vi "Close TDMS File.vi"(8 "error in (no error)":errorcluster caption="错误输入（无错误）", 11 "Log File":refnum<k34> caption="记录文件") -> (0 "error out":errorcluster caption="错误输出", 3 "file path":path caption="记录文件路径")   [LabVIEW 2015]
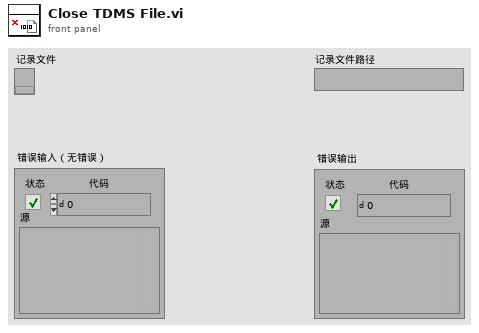
[diagram p1: front panel]
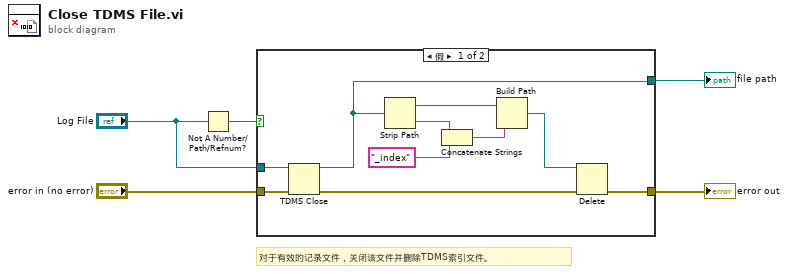
[diagram p0: block diagram]
diagram:
  # "对于有效的记录文件，关闭该文件并删除TDMS索引文件。"
  n1 = Not A Number/Path/Refnum?(number/path/refnum="Log File") -> (NaN/Path/Refnum?=w4:bool)
  n2 = case shown="假" w4 {
    tunnel: [w14 w16] -> w2
    tunnel: "error in (no error)" -> [w8 w16]
    tunnel: "Log File" -> [w7 _]
    tunnel: [w6 _] -> w1
    frame False {
      n3 = TDMS Close(8:w8, 11:w7) -> (0:w9:errorcluster, 3:w6:path)
      n4 = Strip Path(path=w6) -> (stripped path=w12:path, name=w10:string)
      n5 = Concatenate Strings(w10, "_index") -> (w13:string)
      n6 = Build Path(base path=w12, name or relative path=w13) -> (appended path=w15:path)
      n7 = Delete(path (use dialog)=w15, error in=w9) -> (error out=w14:errorcluster)  [unwired: 3 in, 2 out]
    }
    frame True {
    }
  }
  "error out" <- w2
  "file path" <- w1
